vi "BuildRelease_RecompileOpenGDS_RemoveDebugFlag.vi"(11 "VI in":refnum<vi>) -> (3 "VI out":refnum<vi>)   [LabVIEW 2012]
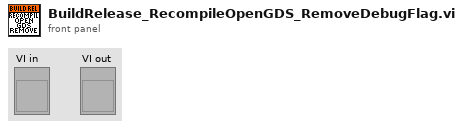
[diagram p1: front panel]
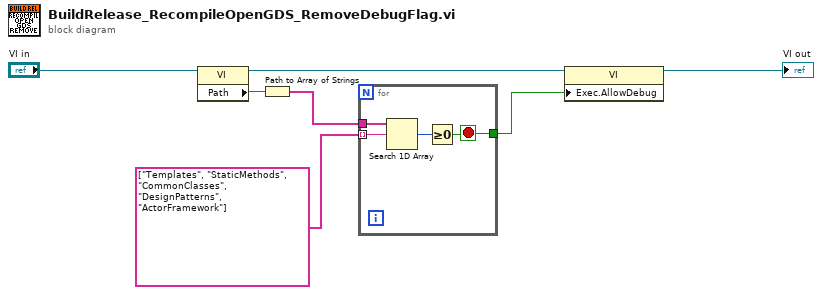
[diagram p0: block diagram]
diagram:
  n1 = property class="VI"(reference="VI in") -> (reference out=w5:refnum<vi>, "Path"=w4:path)  [unwired: 1 in, 1 out]
  n2 = Path to Array of Strings(0:w4) -> (2:w3:string[])  [unwired: 1 out]
  n3 = for {
    tunnel: w3 -> [w11]
    tunnel: string[] ["Templates", "StaticMethods", "CommonClasses", "DesignPatterns", "ActorFramework"] -> [w10] mode=indexing
    tunnel: [w8] -> w1
    stop <- w8 stop-if-true
    n4 = Search 1D Array(1D array=w11, element=w10) -> (index of element=w9:i32)  [unwired: 1 in]
    n5 = Greater Or Equal To 0?(x=w9) -> (x >= 0?=w8:bool)
  }
  n6 = property class="VI"(reference=w5, "Exec.AllowDebug"=w1) -> (reference out=→"VI out":refnum<vi>)  [unwired: 1 in, 1 out]
